vi "Benchmark SV Send  LV2012 - NI Verified - 100 Byte.vi"() -> ()   [LabVIEW 2015]
panel:
  out "100 byte":i32[][](array[numeric])
  in  "Reset":bool
  out "Tries":u32
  out "Average Delay (ms)":dbl
  out "Delay (ms)":u32
  in  "stop":bool
  # "Overview:  Coding that exemplifies how to benchmark the communication of Shared Variables.\nRequirements: LabVIEW 2012 or compatible\nInstructions:\n1.  Run the \"Benchmark SV Receive LV2012 - NI Verified.vi\"\n2. Run this VI\n3. Watch the amount of time it takes to communicate\n4. Stop both VIs"
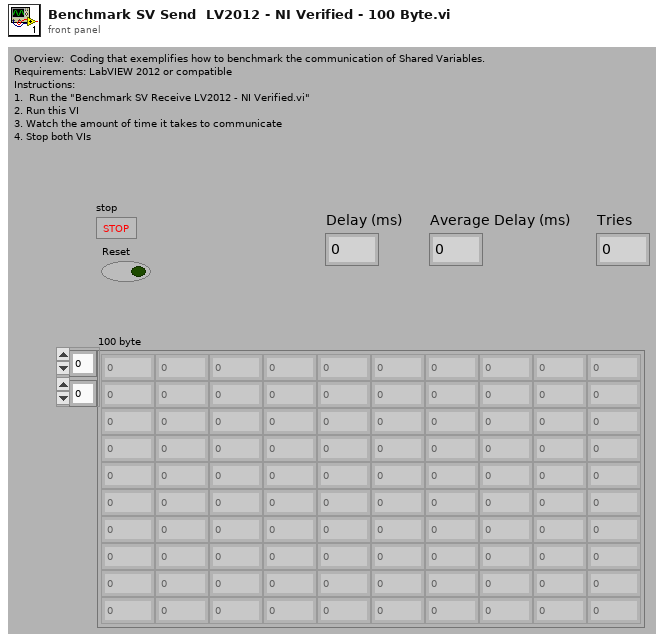
[diagram p1: front panel]
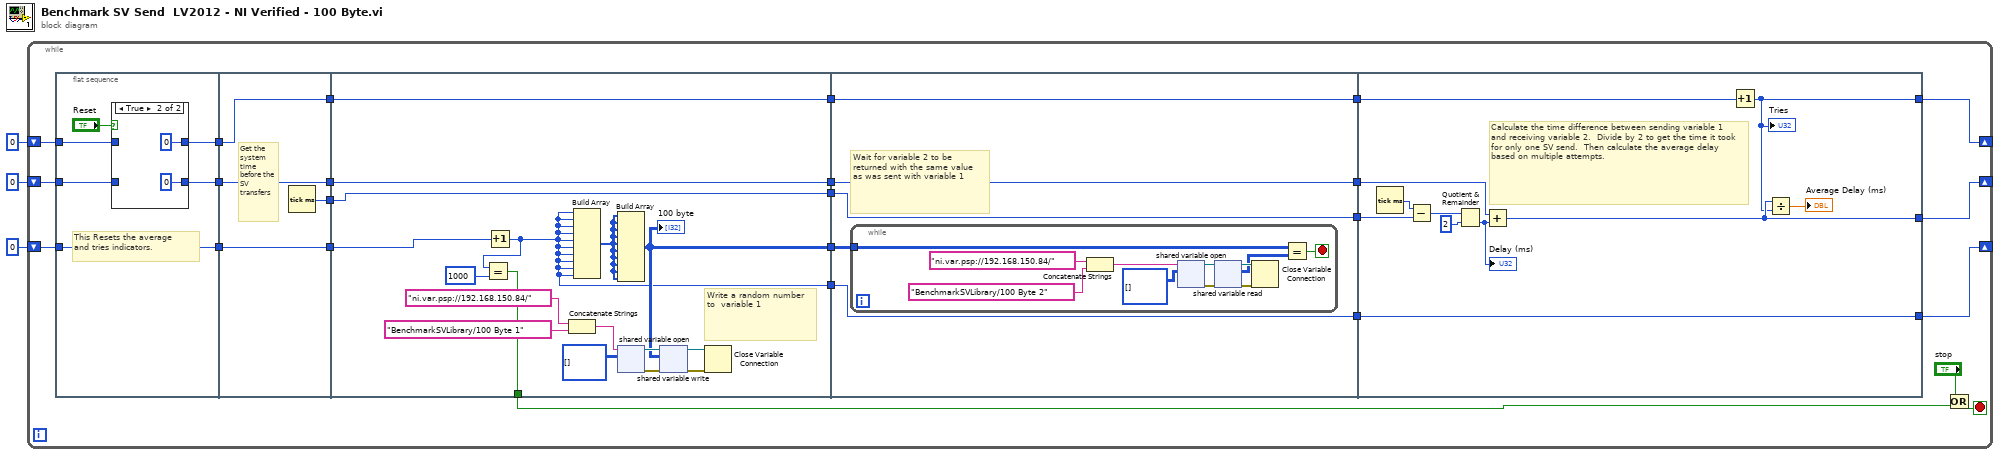
[diagram p0: block diagram]
diagram:
  n1 = while {
    shift-right: [w25] -> _
    shift-left: u32 0 -> [w13]
    shift-right: [w22] -> _
    shift-left: u32 0 -> [w14]
    shift-right: [w7] -> _
    shift-left: 0 -> [w10]
    stop <- w6 stop-if-true
    n2 = flat-sequence {
      tunnel: w13 -> [w34]
      tunnel: [w33] -> w18
      tunnel: [w31] -> w16
      tunnel: w14 -> [w30]
      tunnel: [w29] -> w11
      tunnel: w10 -> [w29]
      tunnel: [w40] -> w19
      tunnel: w18 -> [w42]
      tunnel: [w42] -> w17
      tunnel: w16 -> [w41]
      tunnel: [w41] -> w15
      tunnel: [w39] -> w12
      tunnel: w11 -> [w39]
      tunnel: [w47] -> w28
      tunnel: [w59] -> w27
      tunnel: [w58] -> w23
      tunnel: [w57] -> w20
      tunnel: w19 -> [w59]
      tunnel: w17 -> [w58]
      tunnel: w15 -> [w57]
      tunnel: w12 -> [w49]
      tunnel: [w43] -> w8
      tunnel: [w46] -> w4
      tunnel: w28 -> [w64]
      tunnel: [w63] -> w26
      tunnel: w27 -> [w63]
      tunnel: [w62] -> w24
      tunnel: w23 -> [w62]
      tunnel: [w61] -> w21
      tunnel: w20 -> [w61]
      tunnel: [w60] -> w9
      tunnel: w8 -> [w60]
      tunnel: w26 -> [w85]
      tunnel: [w78] -> w25
      tunnel: w24 -> [w80]
      tunnel: [w77] -> w22
      tunnel: w21 -> [w84]
      tunnel: w9 -> [w76]
      tunnel: [w76] -> w7
      frame #0 {
        # "This Resets the average \nand tries indicators."
        n3 = case shown="True" "Reset" {
          tunnel: [w36 u32 0] -> w33
          tunnel: w34 -> [w36 _]
          tunnel: [w35 u32 0] -> w31
          tunnel: w30 -> [w35 _]
          frame False {
          }
          frame True {
          }
        }
      }
      frame #1 {
        # "Get the system time before the SV transfers"
        n4 = Tick Count (ms)() -> (millisecond timer value=w40:u32)
      }
      frame #2 {
        # "Write a random number to  variable 1"
        n5 = Increment(x=w49) -> (x+1=w43:i32)
        n6 = Equal?(x=w43, y=1000) -> (x = y?=w46:bool)
        n7 = Concatenate Strings("ni.var.psp://192.168.150.84/" ("string"), "BenchmarkSVLibrary/100 Byte 1") -> (w52:string)
        n8 = Build Array(w43, w43, w43, w43, w43, w43, w43, w43, w43, w43) -> (w44:i32[])
        n9 = Build Array(w44, w44, w44, w44, w44, w44, w44, w44, w44, w44) -> (w47:i32[][])
        "100 byte" <- w47
        n10 = shared-variable-open(w52, i32[][] [] ("appended array")) -> (w56:refnum<k21>, w53:errorcluster)  [unwired: 2 in]
        n11 = shared-variable-write(w56, w53, w47) -> (w54:refnum<k21>, w55:errorcluster)
        n12 = Close Variable Connection(8:w55, 11:w54) -> ()  [unwired: 1 out]
      }
      frame #3 {
        # "Wait for variable 2 to be returned with the same value as was sent with variable 1"
        n13 = while {
          tunnel: w64 -> [w66]
          stop <- w75 stop-if-true
          n14 = Concatenate Strings("ni.var.psp://192.168.150.84/" ("string"), "BenchmarkSVLibrary/100 Byte 2") -> (w73:string)
          n15 = shared-variable-open(w73, i32[][] [] ("appended array")) -> (w69:refnum<k21>, w72:errorcluster)  [unwired: 2 in]
          n16 = shared-variable-read(w69, w72) -> (w71:refnum<k21>, w70:errorcluster, w68:i32[][])  [unwired: 1 out]
          n17 = Close Variable Connection(8:w70, 11:w71) -> ()  [unwired: 1 out]
          n18 = Equal?(x=w66, y=w68) -> (x = y?=w75:bool)
        }
      }
      frame #4 {
        # "Calculate the time difference between sending variable 1 and receiving variable 2.  Divide by 2 to get the time it took for only one SV send.  Then calculate the average delay based on multiple attempts."
        n19 = Tick Count (ms)() -> (millisecond timer value=w86:u32)
        n20 = Subtract(x=w86, y=w85) -> (x-y=w83:u32)
        n21 = Quotient & Remainder(x=w83, y=u32 2) -> (floor(x/y)=w81:u32)  [unwired: 1 out]
        "Delay (ms)" <- w81
        n22 = Add(x=w80, y=w81) -> (x+y=w78:u32)
        n23 = Increment(x=w84) -> (x+1=w77:u32)
        "Tries" <- w77
        n24 = Divide(x=w78, y=w77) -> (x/y=→"Average Delay (ms)":dbl)
      }
    }
    n25 = Or(x="stop", y=w4) -> (x .or. y?=w6:bool)
  }
